vi "PointInRect-lv.vi"(1 "P":T2, 2 "R":T1) -> (0 "P contained by R?":bool)   [LabVIEW 2026, in "SDL3.lvlib" / "Rect.lvlib"]
doc: "<B>LV Implementation</B>\nSince the SDL function is inlined, we can't access in the shared library. So it's a LabVIEW implementation of the feature.\n\n<B>Summary</B>\nDetermine whether a point resides inside a rectangle.\n\n<B>Remarks</B>\nA point is considered part of a rectangle if both p and r are not NULL, and p's x and y coordinates are >= to the rectangle's top left corner, and < the rectangle's x+w and y+h. So a 1x1 rectangle considers point (0,0) as \"inside\" and (0,1) as not."
uses:
  Rect.lvlib
  Point--cluster.ctl
  Rect--cluster.ctl
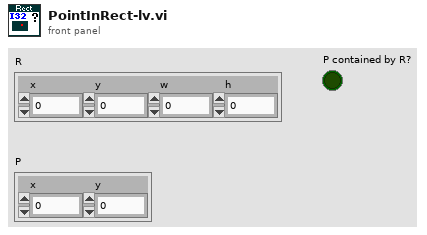
[diagram p1: front panel]
types:
  T1 = typedef "SDL3.lvlib/Rect.lvlib/Rect--cluster.ctl" = cluster{"x":i32, "y":i32, "w":i32, "h":i32}
  T2 = typedef "SDL3.lvlib/Rect.lvlib/Point--cluster.ctl" = cluster{"x":i32, "y":i32}
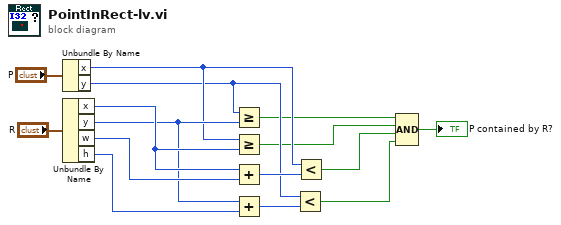
[diagram p0: block diagram]
diagram:
  n1 = Unbundle By Name("P") -> ("x"=w9:i32, "y"=w6:i32)
  n2 = Unbundle By Name("R") -> ("x"=w13:i32, "y"=w11:i32, "w"=w12:i32, "h"=w10:i32)
  n3 = Greater Or Equal?(x=w6, y=w11) -> (x >= y?=w5:bool)
  n4 = Greater Or Equal?(x=w9, y=w13) -> (x >= y?=w4:bool)
  n5 = Add(x=w13, y=w12) -> (x+y=w8:i32)
  n6 = Add(x=w11, y=w10) -> (x+y=w7:i32)
  n7 = Less?(x=w6, y=w7) -> (x < y?=w2:bool)
  n8 = Less?(x=w9, y=w8) -> (x < y?=w3:bool)
  n9 = Compound Arithmetic op=AND(w5, w4, w3, w2) -> (→"P contained by R?":bool)
